vi "Get Server gRPC UEs.vi"(11 "OOP Server in":refnum<class "OCVServer.lvclass">) -> (2 "Server gRPC UEs":T1, 3 "OOP Server out":refnum<class "OCVServer.lvclass">)   [LabVIEW 2019, in "OCVServer.lvlib" / "OCVServer.lvclass"]
uses:
  OCVServer.lvclass
  typeDefs/Server gRPC UEs.ctl
  gRPC lvSupport/Server API/typeDefs/gRPCId Cluster UE.ctl
  gRPC lvSupport/Server API/typeDefs/gRPCId Cluster.ctl
  gRPC lvSupport/Server API/typeDefs/grpcId.ctl
  OCVServer.lvclass/OCVServer.ctl
  gRPC lvSupport/gprc-lvsupport.lvlib
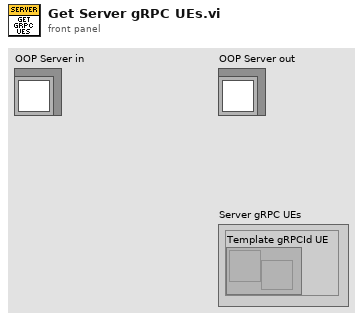
[diagram p1: front panel]
types:
  T1 = typedef "OCVServer.lvlib/OCVServer.lvclass/Server gRPC UEs.ctl" = cluster{"Template gRPCId UE":T2}
  T2 = typedef "OCVServer.lvlib/gprc-lvsupport.lvlib/gRPCId Cluster UE.ctl" = refnum<user-event>
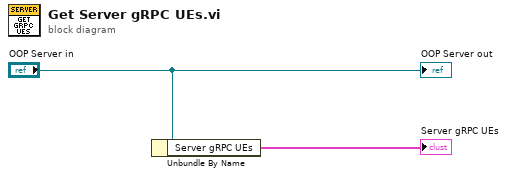
[diagram p0: block diagram]
diagram:
  n1 = Unbundle By Name("OOP Server in") -> ("Server gRPC UEs"=→"Server gRPC UEs":T1)
  "OOP Server out" <- "OOP Server in"
